vi "assignment2.vi"() -> ()   [LabVIEW 2020]
panel:
  in  "length (rest)":i32=9
  out "substring":string
  out "replaced substring":string
  out "result string 2":string
  in  "length (len. of substring)":i32=6
  in  "offset (0) 3":i32=6
  in  "substring (\"\")":string="I"
  in  "string 2":string="Hello Vijeet want to play "
  in  "offset (0) 2":i32=2
  in  "string":string="I am Vijeet Khadilkar"
  out "error out":errorcluster
  out "offset past replacement":i32
  out "number of replacements":i32
  out "result string":string
  in  "replace string (\"\")":string="I"
  in  "offset (0)":i32=8
  in  "search string":string="Vijeet"
  in  "input string":string="Vijeet done the work. Vijeet have cook the food. Vijeet go to Nagpur."
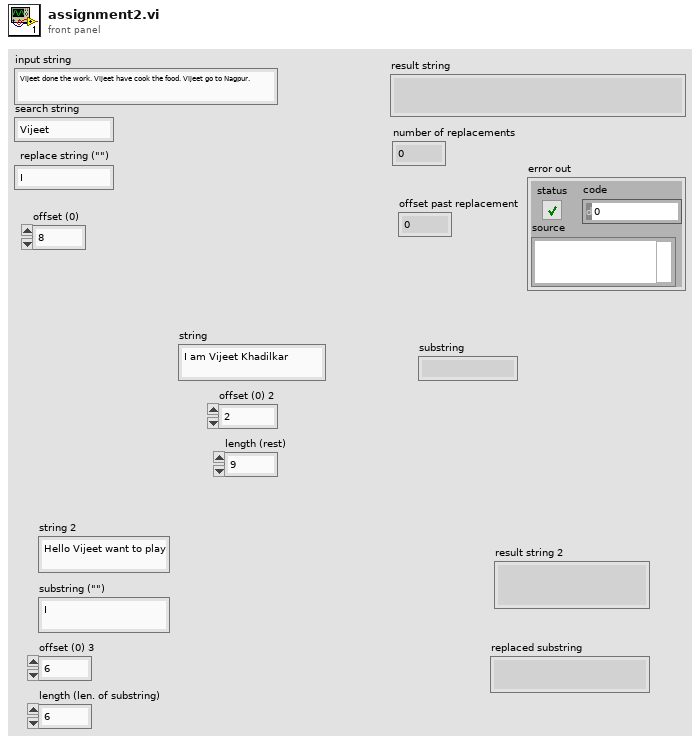
[diagram p1: front panel]
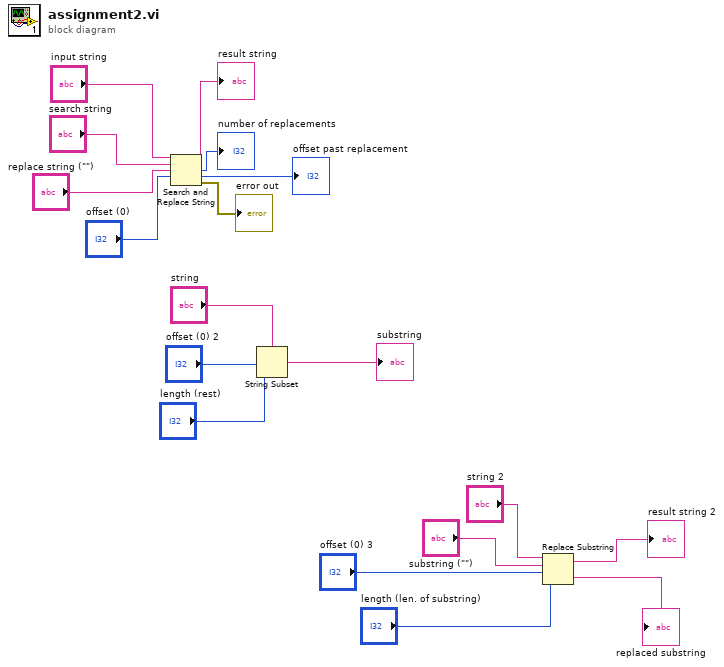
[diagram p0: block diagram]
diagram:
  n1 = Search and Replace String(input string="input string", search string="search string", replace string="replace string (\"\")", offset="offset (0)") -> (result string=→"result string":string, number of replacements=→"number of replacements":i32, offset past replacement=→"offset past replacement":i32, error out=→"error out":errorcluster)  [unwired: 4 in]
  n2 = String Subset(string="string", offset (0)="offset (0) 2", length (rest)="length (rest)") -> (substring=→"substring":string)
  n3 = Replace Substring(2:"length (len. of substring)", 3:"offset (0) 3", 4:"substring (\"\")", 5:"string 2") -> (0:→"replaced substring":string, 1:→"result string 2":string)
